vi "Configure Mode.vi"(7 "error in (no error)":errorcluster, 9 "Mode (0: FLOW)":u16(ring) items=["FLOW", "RAMP"], 10 "VISA resource name":refnum<visa-resource-name>) -> (0 "error out":errorcluster, 3 "VISA resource name out":refnum<visa-resource-name>)   [LabVIEW 2018]
panel:
  out "read buffer":string
  out "resulting string":string
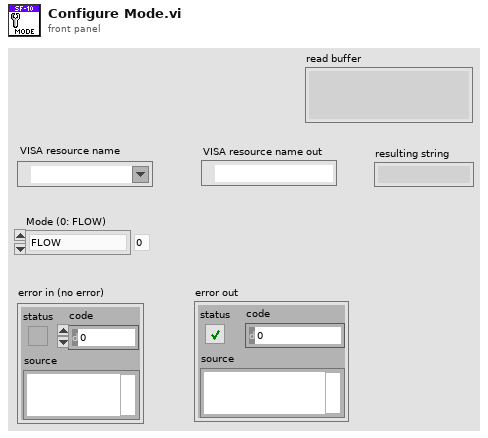
[diagram p1: front panel]
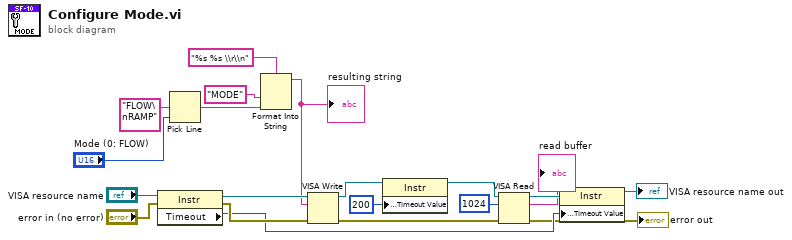
[diagram p0: block diagram]
diagram:
  n1 = property class="Instr"(reference="VISA resource name", error in="error in (no error)") -> (reference out=w16:refnum<visa-resource-name>, error out=w14:errorcluster, "Timeout"=w8:u32)
  n2 = Pick Line(multi-line string="FLOW\nRAMP", line index="Mode (0: FLOW)") -> (output string=w3:string)  [unwired: 1 in]
  n3 = Format Into String(format string="%s %s \\r\\n", "MODE" ("initial string"), w3) -> (resulting string=w15:string)  [unwired: 2 in, 1 out]
  "resulting string" <- w15
  n4 = VISA Write(VISA resource name=w16, write buffer=w15, error in (no error)=w14) -> (VISA resource name out=w12:refnum<visa-resource-name>, error out=w7:errorcluster)  [unwired: 1 out]
  n5 = property class="Instr"(reference=w12, "General Settings:Timeout Value"=u32 200) -> (reference out=w10:refnum<visa-resource-name>)  [unwired: 1 in, 1 out]
  n6 = VISA Read(VISA resource name=w10, byte count=u32 1024, error in (no error)=w7) -> (VISA resource name out=w9:refnum<visa-resource-name>, read buffer=→"read buffer":string, error out=→"error out":errorcluster)  [unwired: 1 out]
  n7 = property class="Instr"(reference=w9, "General Settings:Timeout Value"=w8) -> (reference out=→"VISA resource name out":refnum<visa-resource-name>)  [unwired: 1 in, 1 out]
